vi "TX-UDP-DE.vi"(0 "Transmitter port number":u16, 5 "IP address":string, 7 "Receiver Port number":u16, 9 "channel":T1, 11 "error in (no error)":errorcluster) -> (4 "Loop iterations":i32, 6 "Transmitter port":u16, 8 "error out":errorcluster)   [LabVIEW 2017]
uses:
  <extravilib>/ChannelInstances/Tag-dbl/))Channel.ctl
  <extravilib>/ChannelInstances/Tag-dbl/Read With Abort.vi
  <extravilib>/ChannelInstances/Tag-dbl/EndpointRead.vi
  <extravilib>/ChannelInstances/Tag-dbl.lvlib
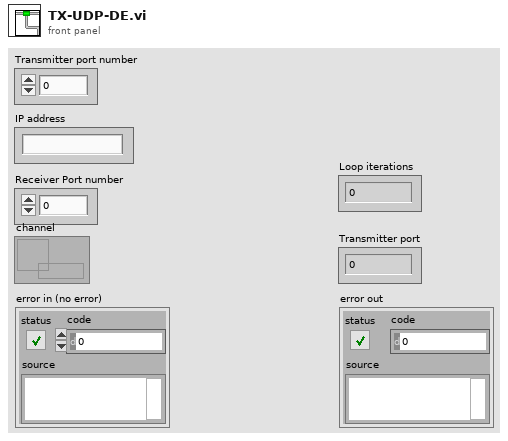
[diagram p1: front panel]
types:
  T1 = typedef "Tag-dbl.lvlib/))Channel.ctl" = refnum<queue>
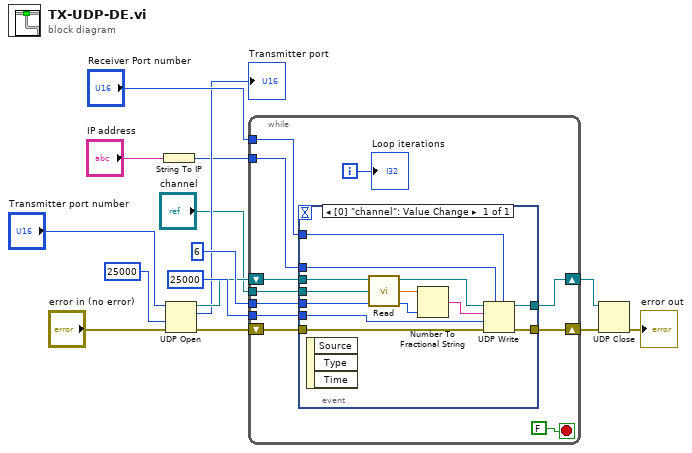
[diagram p0: block diagram]
diagram:
  n1 = String To IP(1:"IP address") -> (0:w3:u32)
  n2 = UDP Open(8:"error in (no error)", 9:25000 ("timeout ms (25000)"), 11:"Transmitter port number") -> (port=w9:refnum<k16>, 0:w10:errorcluster, 2:→"Transmitter port":u16)  [unwired: 2 in]
  n3 = while {
    tunnel: 25000 ("timeout ms (25000)") -> [w26]
    tunnel: "Receiver Port number" -> [w25]
    tunnel: w3 -> [w24]
    tunnel: i16 6 ("precision (6)") -> [w23]
    shift-right: [w19] -> w7
    shift-left: w10 -> [w22]
    shift-right: [w20] -> w8
    shift-left: w9 -> [w21]
    tunnel: "channel" -> [w16]
    i -> [w18]
    stop <- FALSE stop-if-true
    n4 = event shown="[0] \"channel\": Value Change" {
      selector: _ -> [_]
      dyn-events: _ -> [_]
      timeout: _ -> [_]
      tunnel: w26 -> [w37]
      tunnel: w25 -> [w36]
      tunnel: w24 -> [w35]
      tunnel: [w34] -> w19
      tunnel: [w33] -> w20
      tunnel: w23 -> [w31]
      tunnel: w22 -> [w30]
      tunnel: w21 -> [w29]
      tunnel: w16 -> [w27]
      event Value Change {
        n5 = event-data() -> ()  [unwired: 1 in, 3 out]
        n6 = call <extravilib>:"Read.vi"("channel"=w27) -> ("element"=w28:dbl)  [unwired: 1 in, 1 out]
        n7 = Number To Fractional String(number=w28, precision (6)=w31) -> (F-format string=w32:string)  [unwired: 2 in]
        n8 = UDP Write(address=w35, port or service name=w36, connection ID=w29, data in=w32, 8:w30, 9:w37) -> (error out=w34:errorcluster, 3:w33:refnum<k16>)
      }
    }
    "Loop iterations" <- w18
  }
  n9 = UDP Close(connection ID=w8, 8:w7) -> (error out=→"error out":errorcluster)  [unwired: 1 out]
